vi "mod_Envelope Detection.vi"(0 "input data":waveform(dbl)={"t0"=timestamp(0 s since 1904-01-01), "dt"=0.0, "Y"=[]}, 1 "RC":dbl=0.16 format="%.2f", 12 "SC":dbl=0.00025316455696202533 format="%.6f") -> (4 "QP Output":dbl[](array[numeric])=[0.0065936346025232614, 0.0065923160074666575, 0.006590997676102695, 0.00658967960837864, 0.006588361804241771, 0.006587044263639375, 0.0065857269865187505, 0.006584409972827206, 0.006583093222512062, 0.006581776735520647, 0.0065804605118003024, 0.006579144551298379, 0.006577828853962239, 0.006576513419739253, 0.006575198248576805, 0.006573883340422288, 0.0065725686952231065, 0.006571254312926673, 0.006569940193480413, 0.006568626336831761, 0.006567312742928164, 0.006565999411717077, 0.006564686343145968, 0.006563373537162314, 0.006562060993713602, 0.00656074871274733, 0.006559436694211007, 0.0065581249380521536, 0.006556813444218298, 0.006555502212656982, 0.006554191243315755, 0.006552880536142178, 0.006551570091083823, 0.006550259908088273, 0.006548949987103121, 0.006547640328075969, 0.00654633093095443, 0.00654502179568613, 0.006543712922218703, 0.0065424043104997925, 0.006541095960477056, 0.0065397878720981585, 0.006538480045310777, 0.006537172480062598, 0.006535865176301319, 0.006534558133974648, 0.006533251353030304, 0.006531944833416015, 0.00653063857507952, 0.0065293325779685685, 0.006528026842030921, 0.0065267213672143476, 0.00652541615346663, 0.00652411120073556, 0.006522806508968939, 0.006521502078114578, 0.006520197908120302, 0.006518893998933943, 0.006517590350503344, 0.006516286962776361, 0.006514983835700857, 0.006513680969224707, 0.006512378363295797, 0.006511076017862023, 0.00650977393287129, 0.0065084721082715145, 0.006507170544010625, 0.006505869240036558, 0.006504568196297262, 0.006503267412740694, 0.006501966889314824, 0.00650066662596763, 0.006499366622647102, 0.00649806687930124, 0.006496767395878053, 0.0064954681723255634, 0.006494169208591802, 0.006492870504624809, 0.006491572060372638, 0.006490273875783349, 0.0064889759508050164, 0.006487678285385723, 0.006486380879473562, 0.006485083733016636, 0.006483786845963061, 0.006482490218260961, 0.006481193849858471, 0.0064798977407037345, 0.006478601890744909, 0.00647730629993016, 0.006476010968207664, 0.0064747158955256075, 0.006473421081832188, 0.006472126527075612, 0.0064708322312040985, 0.006469538194165875, 0.00646824441590918, 0.006466950896382263, 0.006465657635533382, 0.006464364633310808, 0.00646307188966282, 0.006461779404537708, 0.006460487177883774, 0.006459195209649327, 0.006457903499782689, 0.006456612048232193, 0.0064553208549461795, 0.006454029919873001, 0.006452739242961019, 0.006451448824158609, 0.006450158663414152, 0.006448868760676043, 0.006447579115892685, 0.006446289729012493, 0.00644500059998389, 0.006443711728755313, 0.006442423115275205, 0.006441134759492023, 0.006439846661354233, 0.006438558820810309, 0.006437271237808739, 0.006435983912298019, 0.0064346968442266575, 0.00643341003354317, 0.006432123480196084, 0.006430837184133939, 0.006429551145305282, 0.006428265363658672, 0.0064269798391426766, 0.006425694571705876, 0.0064244095612968595, 0.006423124807864226, 0.006421840311356585, 0.0064205560717225585, 0.006419272088910775, 0.006417988362869876, 0.006416704893548513, 0.0064154216808953455, 0.006414138724859047, 0.006412856025388298, 0.006411573582431791, 0.006410291395938228, 0.006409009465856322, 0.006407727792134795, 0.00640644637472238, 0.006405165213567822, 0.006403884308619873, 0.006402603659827298, 0.006401323267138869, 0.006400043130503371, 0.006398763249869601, 0.006397483625186361, 0.006396204256402467, 0.006394925143466744, 0.0063936462863280275, 0.006392367684935164, 0.006391089339237007, 0.006389811249182426, 0.0063885334147202955, 0.006387255835799502, 0.006385978512368943, 0.006384701444377525, 0.0063834246317741655, 0.006382148074507793, 0.006380871772527344, 0.006379595725781766, 0.0063783199342200185, 0.006377044397791069, 0.006375769116443897, 0.00637449409012749, 0.006373219318790847, 0.006371944802382979, 0.0063706705408529025, 0.006369396534149649, 0.006368122782222258, 0.0063668492850197786, 0.006365576042491271, 0.006364303054585807, 0.006363030321252466, 0.006361757842440339, 0.006360485618098525, 0.006359213648176138, 0.006357941932622297, 0.006356670471386134, 0.006355399264416792, 0.0063541283116634205, 0.006352857613075183, 0.00635158716860125, 0.006350316978190804, 0.0063490470417930395, 0.006347777359357157, 0.006346507930832369, 0.0063452387561679, 0.006343969835312982, 0.006342701168216857, 0.00634143275482878, 0.006340164595098015, 0.006338896688973834, 0.006337629036405522, 0.006336361637342372, 0.006335094491733688, 0.0063338275995287845, 0.006332560960676986, 0.006331294575127627, 0.006330028442830052, 0.006328762563733615, 0.006327496937787682, 0.006326231564941627, 0.0063249664451448355, 0.006323701578346702, 0.0063224369644966335, 0.006321172603544044, 0.0063199084954383596, 0.006318644640129016, 0.006317381037565458, 0.006316117687697143, 0.006314854590473536, 0.006313591745844114, 0.006312329153758363, 0.006311066814165779, 0.006309804727015867, 0.006308542892258146, 0.006307281309842141, 0.00630601997971739, 0.006504885190669998, 0.006703219941249714, 0.006701879431316926, 0.006700539189459316, 0.006699199215623274, 0.006697859509755202, 0.006696520071801511, 0.006695180901708624, 0.006693841999422974, 0.006692503364891004, 0.00669116499805917, 0.006689826898873937, 0.006688489067281781, 0.006687151503229189, 0.0066858142066626575, 0.006684477177528695, 0.0066831404157738205, 0.006681803921344564, 0.006680467694187465, 0.006679131734249074, 0.006677796041475954, 0.0066764606158146765, 0.0066751254572118245, 0.006673790565613991, 0.006672455940967782, 0.006671121583219811, 0.006669787492316705, 0.006668453668205098, 0.00666712011083164, 0.006665786820142987, 0.006664453796085808, 0.006663121038606782, 0.006661788547652598, 0.0066604563231699564, 0.006659124365105569, 0.006657792673406156, 0.006656461248018452, 0.0066551300888891985, 0.00665379919596515, 0.006652468569193069, 0.006651138208519733, 0.0066498081138919255, 0.006648478285256444, 0.006647148722560094, 0.006645819425749694, 0.006644490394772072, 0.006643161629574066, 0.0066418331301025275, 0.006640504896304314, 0.006639176928126297, 0.0066378492255153585, 0.00663652178841839, 0.006635194616782294, 0.006633867710553984, 0.006632541069680383, 0.006631214694108425, 0.006629888583785056, 0.006628562738657232, 0.006627237158671918, 0.006625911843776091, 0.006624586793916738, 0.006623262009040858, 0.006621937489095459, 0.006620613234027561, 0.006619289243784194, 0.006617965518312396, 0.006616642057559221, 0.006615318861471728, 0.006613995929996991, 0.006612673263082092, 0.006611350860674124, 0.006610028722720192, 0.00660870684916741, 0.006607385239962902, 0.006606063895053805, 0.0066047428143872645, 0.006603421997910437, 0.006602101445570491, 0.006600781157314603, 0.006599461133089963, 0.006598141372843769, 0.006596821876523231, 0.0065955026440755685, 0.006594183675448013, 0.006592864970587805, 0.006591546529442197, 0.006590228351958451, 0.00658891043808384] format="%.2f", 14 "QP Last Value":dbl=0.00658891043808384 format="%.2f")   [LabVIEW 2020, in "niDMT.lvlib"]
uses:
  <vilib>/addons/Modulation/niDMT.lvlib
panel:
  in  "QPPrevious":dbl=0.00659495346132525 format="%.2f"
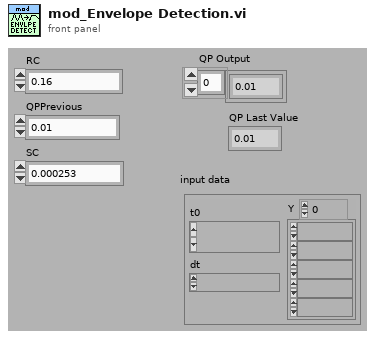
[diagram p1: front panel]
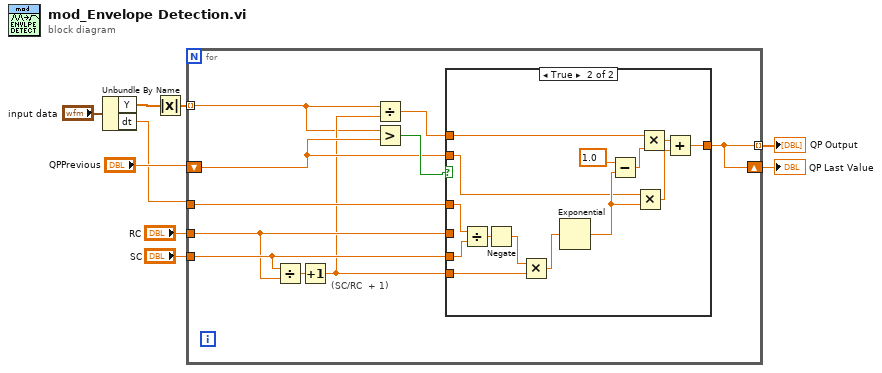
[diagram p0: block diagram]
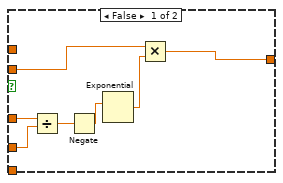
[diagram p2: hidden frame]
diagram:
  n1 = Unbundle By Name("input data") -> ("Y"=w2:dbl[], "dt"=w1:dbl)
  n2 = Absolute Value(x=w2) -> (abs(x)=w4:dbl[])
  n3 = for {
    shift-right: [w10] -> w7
    shift-left: "QPPrevious" -> [w18]
    tunnel: "RC" -> [w15]
    tunnel: w4 -> [w11] mode=indexing
    tunnel: w1 -> [w17]
    tunnel: [w10] -> w8 mode=indexing
    tunnel: "SC" -> [w16]
    # "(SC/RC  + 1)"
    n4 = Divide(x=w16, y=w15) -> (x/y=w14:dbl)
    n5 = Increment(x=w14) -> (x+1=w12:dbl)
    n6 = Divide(x=w11, y=w12) -> (x/y=w13:dbl)
    n7 = Greater?(x=w11, y=w18) -> (0:w19:bool)
    n8 = case shown="True" w19 {
      tunnel: w13 -> [_ w38]
      tunnel: [w21 w34] -> w10
      tunnel: w15 -> [w25 _]
      tunnel: w17 -> [w26 w32]
      tunnel: w18 -> [w20 w27]
      tunnel: w16 -> [_ w31]
      tunnel: w12 -> [_ w33]
      frame False {
        n9 = Divide(x=w26, y=w25) -> (x/y=w24:dbl)
        n10 = Negate(x=w24) -> (-x=w23:dbl)
        n11 = Exponential(1:w23) -> (0:w22:dbl)
        n12 = Multiply(x=w20, y=w22) -> (x*y=w21:dbl)
      }
      frame True {
        n13 = Divide(x=w32, y=w31) -> (x/y=w40:dbl)
        n14 = Negate(x=w40) -> (-x=w29:dbl)
        n15 = Multiply(x=w29, y=w33) -> (x*y=w28:dbl)
        n16 = Exponential(1:w28) -> (0:w37:dbl)
        n17 = Subtract(x=1.0, y=w37) -> (x-y=w30:dbl)
        n18 = Multiply(x=w27, y=w37) -> (x*y=w36:dbl)
        n19 = Multiply(x=w38, y=w30) -> (x*y=w35:dbl)
        n20 = Add(x=w35, y=w36) -> (x+y=w34:dbl)
      }
    }
  }
  "QP Output" <- w8
  "QP Last Value" <- w7
